vi "Check if configuration files exist.vi"(8 "error in (no error)":errorcluster, 11 "AOTFBase in":refnum<class "AOTF.lvclass">) -> (0 "error out":errorcluster, 2 "configuration file exists?":bool, 3 "AOTFBase out":refnum<class "AOTF.lvclass">)   [LabVIEW 2012]
doc: "Checks whether all required configuration files for the component exist."
uses:
  <vilib>/Distrio/Murmex/Murmex/Murmex.lvclass
  AOTF.lvclass
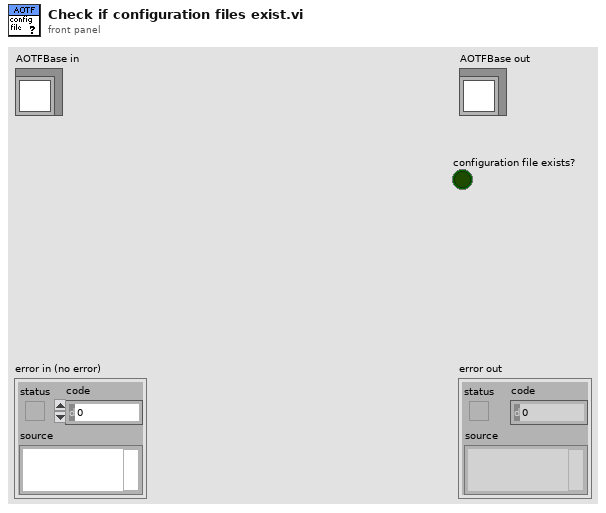
[diagram p1: front panel]
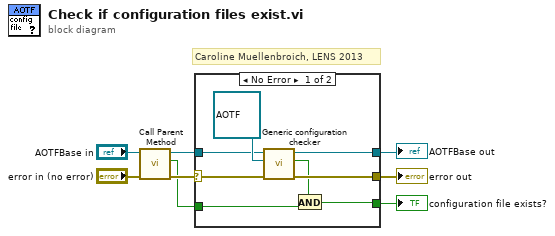
[diagram p0: block diagram]
diagram:
  # "Caroline Muellenbroich, LENS 2013"
  n1 = call-parent "Call Parent Method"("error in (no error)"="error in (no error)", "MurmexBase in"="AOTFBase in") -> ("error out"=w6:errorcluster, "configuration file exists?"=w2:bool, "MurmexBase out"=w4:refnum<class "AOTF.lvclass">)  [unwired: 7 in]
  n2 = case shown="No Error" w6 {
    selector: w6 -> [w16 w18]
    tunnel: [w15 w18] -> w5
    tunnel: w4 -> [w13 w19]
    tunnel: [w12 w19] -> w3
    tunnel: w2 -> [w10 w17]
    tunnel: [w9 w17] -> w1
    frame No Error {
      n3 = call <vilib>:"Generic configuration checker.vi"("error in (no error)"=w16, 10:refnum<class "AOTF.lvclass"> refnum ("AOTF"), "Murmex in"=w13) -> ("error out"=w15:errorcluster, "configuration file exists?"=w11:bool, "Murmex out"=w12:refnum<class "AOTF.lvclass">)  [unwired: 6 in]
      n4 = And(x=w11, y=w10) -> (x .and. y?=w9:bool)
    }
    frame Error {
    }
  }
  "error out" <- w5
  "AOTFBase out" <- w3
  "configuration file exists?" <- w1
